vi "Image.vi"(2 "XRef":refnum<vi>, 3 "State In":T1={"Input Type"=variant(path path ""), "Terminals"=[]}) -> (0 "Image":picture)   [LabVIEW 2015, in "Await.xnode"]
doc: "This ability VI is used to describe your XNode's appearance. The origin of Image corresponds to the top-left corner of your XNode. The bounds of your XNode are used to crop this image. If you want LabVIEW to update your image, you need to inform it through the UpdateImage or UpdateImageAndBounds replies. Any areas where you do not draw are transparent, so regions intended to appear white should be explicitly drawn.\n \n Remember to localize any strings that are part of your image.\n\nDefault behavior: None.\n\nThis ability does not provide UI and OS messages are not handled."
uses:
  Await.xnode
  State.ctl
  <vilib>/picture/picture.llb/imagedata.ctl
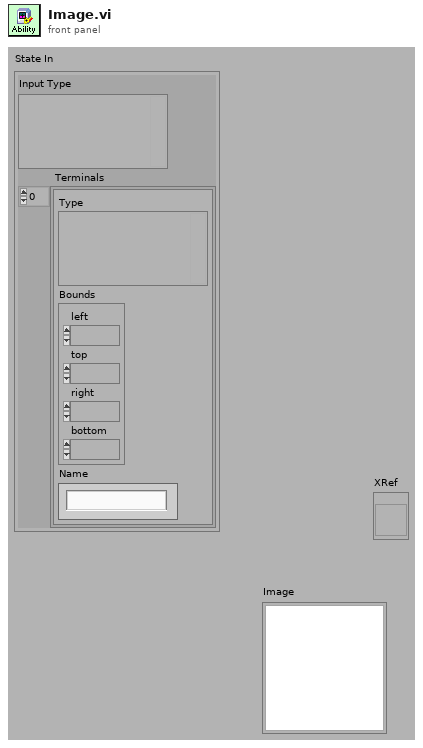
[diagram p1: front panel]
types:
  T1 = typedef "Await.xnode/State.ctl" = cluster{"Input Type":variant, "Terminals":cluster{"Type":variant, "Bounds":cluster{"left":i16, "top":i16, "right":i16, "bottom":i16}, "Name":string}[]}
  T2 = typedef "imagedata.ctl" = cluster{"image type":i32, "image depth":i32, "image":u8[], "mask":u8[], "colors":u32[], "Rectangle":cluster{"left":i16, "top":i16, "right":i16, "bottom":i16}}
  T3 = cluster{"Type":variant, "Bounds":cluster{"left":i16, "top":i16, "right":i16, "bottom":i16}, "Name":string}[]
  T4 = cluster{"left":i16, "top":i16, "right":i16, "bottom":i16}
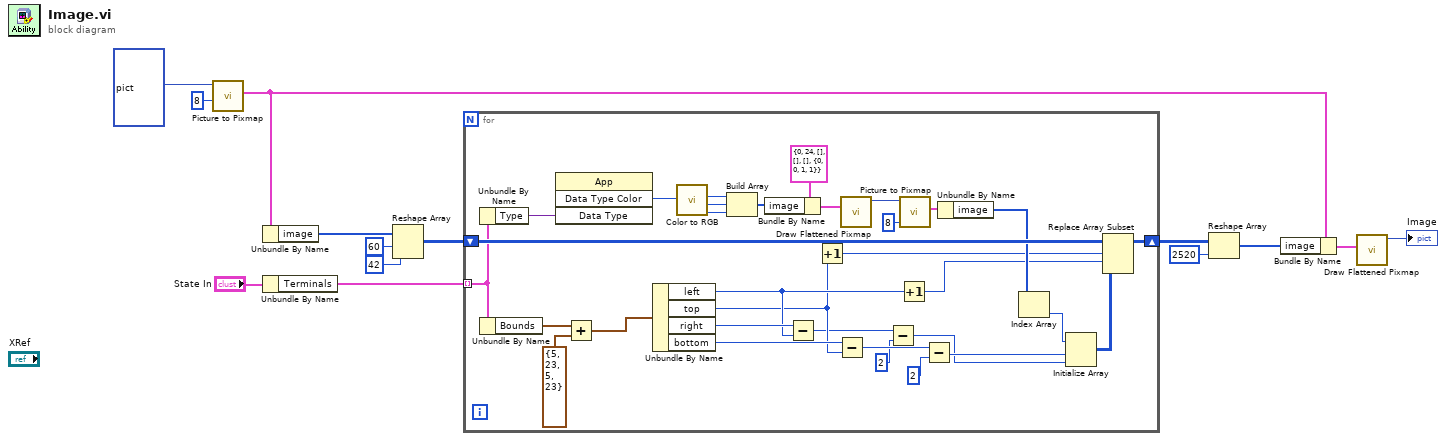
[diagram p0: block diagram]
diagram:
  n1 = call <vilib>:"Picture to Pixmap.vi"("depth"=8, "picture"=picture bytes[7950] ("Image")) -> ("image data"=w14:T2)  [unwired: 8 in, 1 out]
  n2 = Unbundle By Name(w14) -> ("image"=w6:u8[])
  n3 = Unbundle By Name("State In") -> ("Terminals"=w4:T3)
  n4 = Reshape Array(w6, 60 ("dimension size"), 42 ("dimension size")) -> (w9:u8[][])
  n5 = for {
    shift-right: [w45] -> w8
    shift-left: w9 -> [w46]
    tunnel: w4 -> [w38] mode=indexing
    n6 = Unbundle By Name(w38) -> ("Type"=w36:variant)
    n7 = Unbundle By Name(w38) -> ("Bounds"=w33:T4)
    n8 = invoke class="App" method="Data Type Color"("Data Type"=w36) -> ("Data Type Color"=w32:u32)  [unwired: 3 in, 3 out]
    n9 = Add(x=w33, y=T4 {"left"=5, "top"=23, "right"=5, "bottom"=23}) -> (x+y=w37:T4)
    n10 = Unbundle By Name(w37) -> ("left"=w43:i16, "top"=w41:i16, "right"=w44:i16, "bottom"=w42:i16)
    n11 = call <vilib>:"Color to RGB.vi"("Color"=w32) -> ("R"=w31:u8, "G"=w30:u8, "B"=w29:u8)  [unwired: 1 out]
    n12 = Build Array(w31, w30, w29) -> (w28:u8[])
    n13 = Bundle By Name(cluster=T2 {"image type"=0, "image depth"=24, "image"=[], "mask"=[], "colors"=[], "Rectangle"={"left"=0, "top"=0, "right"=1, "bottom"=1}} ("image data"), "image"=w28) -> (w25:T2)
    n14 = Subtract(x=w44, y=w43) -> (x-y=w18:i16)
    n15 = Increment(x=w41) -> (x+1=w16:i16)
    n16 = Subtract(x=w42, y=w41) -> (x-y=w35:i16)
    n17 = call <vilib>:"Draw Flattened Pixmap.vi"("image data"=w25) -> ("new picture"=w26:picture)  [unwired: 8 in]
    n18 = Subtract(x=w18, y=i16 2 ("x")) -> (x-y=w17:i16)
    n19 = Increment(x=w43) -> (x+1=w15:i16)
    n20 = call <vilib>:"Picture to Pixmap.vi"("depth"=8, "picture"=w26) -> ("image data"=w24:T2)  [unwired: 8 in, 1 out]
    n21 = Subtract(x=w35, y=i16 2 ("x")) -> (x-y=w21:i16)
    n22 = Unbundle By Name(w24) -> ("image"=w23:u8[])
    n23 = Index Array(array=w23) -> (element=w22:u8)  [unwired: 1 in]
    n24 = Initialize Array(w22, w21, w17) -> (w40:u8[][])
    n25 = Replace Array Subset(array=w46, new element=w40, index (row)=w16, index (col)=w15) -> (w45:u8[][])
  }
  n26 = Reshape Array(w8, 2520 ("dimension size")) -> (w5:u8[])
  n27 = Bundle By Name(cluster=w14, "image"=w5) -> (w3:T2)
  n28 = call <vilib>:"Draw Flattened Pixmap.vi"("image data"=w3) -> ("new picture"=→"Image":picture)  [unwired: 8 in]
